vi "Send FlushAckMsg.vi"(8 "error in (no error)":errorcluster, 10 "appenderID":string, 11 "Enqueuer in":refnum<class "Message Enqueuer.lvclass">) -> (0 "error out":errorcluster, 3 "Enqueuer out":refnum<class "Message Enqueuer.lvclass">)   [LabVIEW 2026, in "Lumberjack.lvlib" / "FlushAckMsg.lvclass"]
uses:
  FlushAckMsg.lvclass
  FlushAckMsg.lvclass/FlushAckMsg.ctl
  C:/Program Files (x86)/National Instruments/LabVIEW 2026/vi.lib/ActorFramework/Message/Message.lvclass
  C:/Users/dallis/OneDrive - Velico Medical/Documents/Personal/LabVIEW Coding Projects/Lumberjack/src/Core/Messages/FlushAckMsg.lvclass/FlushAckMsg.lvclass
  <vilib>/ActorFramework/Message Enqueuer/Message Enqueuer.lvclass
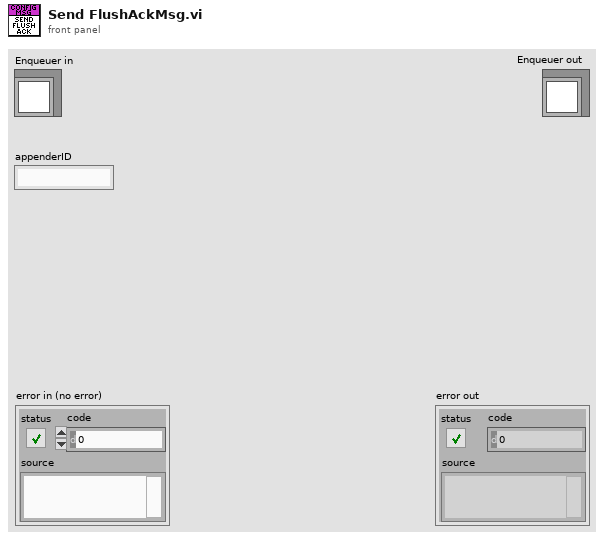
[diagram p1: front panel]
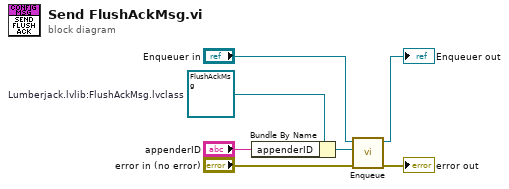
[diagram p0: block diagram]
diagram:
  w3 = refnum<class "FlushAckMsg.lvclass"> refnum  # Lumberjack.lvlib:FlushAckMsg.lvclass
  n1 = Bundle By Name(cluster=w3, "appenderID"="appenderID") -> (w2:refnum<class "FlushAckMsg.lvclass">)
  n2 = call <vilib>:"Enqueue.vi"("error in (no error)"="error in (no error)", "Message"=w2, "Message Enqueuer in"="Enqueuer in") -> ("error out"=→"error out":errorcluster, "Message Enqueuer out"=→"Enqueuer out":refnum<class "Message Enqueuer.lvclass">)  [unwired: 7 in]
